vi "SMC_GetError.vi"(8 "error in (no error)":errorcluster) -> (0 "error out":errorcluster, 1 "ErrorText":string, 3 "Answer":string)   [LabVIEW 2015]
uses:
  SMC_SubVIs.llb/SMC_ManagerMode.ctl
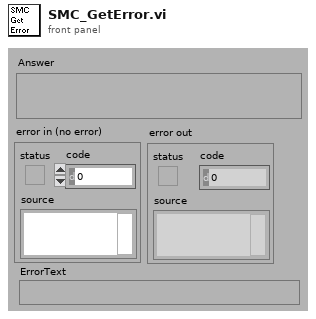
[diagram p1: front panel]
types:
  T1 = typedef "SMC_ManagerMode.ctl" = enum16{"Init", "Get", "SetPosition", "SetStatus", "SetMoving", "SetControllerNr"}
  T2 = typedef "SMC Paras.ctl" = cluster{"VENUS Language":T3, "Number of Axis":u8, "Controller Nr":u8, "Simulation":bool}
  T3 = typedef "VENUSNr.ctl" = enum16{"VENUS 2", "VENUS 1"}
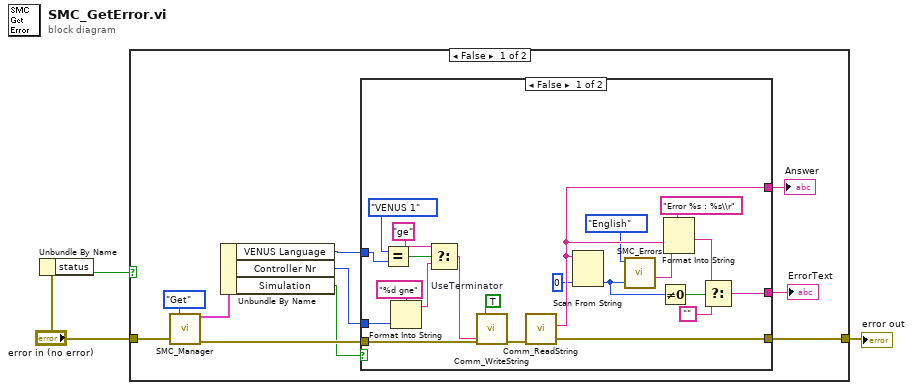
[diagram p0: block diagram]
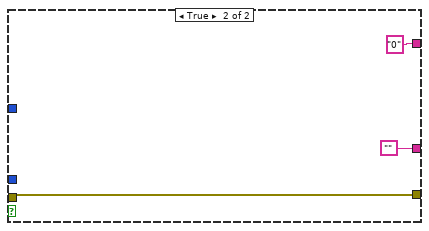
[diagram p2: hidden frame]
diagram:
  n1 = Unbundle By Name("error in (no error)") -> ("status"=w2:bool)
  n2 = case shown="False" w2 {
    tunnel: "error in (no error)" -> [w9 w39]
    tunnel: [w10 w39] -> w1
    frame False {
      n3 = call "SMC_Manager.vi"("Mode"=SMC_ManagerMode."Get", "error in (no error)"=w9) -> ("SMC Parameter Out"=w7:T2, "error out"=w8:errorcluster)  [unwired: 9 in, 3 out]
      n4 = Unbundle By Name(w7) -> ("VENUS Language"=w5:T3, "Controller Nr"=w6:u8, "Simulation"=w4:bool)
      n5 = case shown="False" w4 {
        tunnel: [w35 ""] -> w12
        tunnel: [w34 "0" ("Answer")] -> w11
        tunnel: [w33 w36] -> w10
        tunnel: w8 -> [w32 w36]
        tunnel: w5 -> [w21 _]
        tunnel: w6 -> [w15 _]
        frame False {
          w14 = TRUE  # UseTerminator
          n6 = Equal?(x=enum16{"VENUS 2", "VENUS 1"}."VENUS 1", y=w21) -> (x = y?=w22:bool)
          n7 = Format Into String(format string="%d gne" ("Format String"), w15) -> (resulting string=w16:string)  [unwired: 2 in, 1 out]
          n8 = Select(t="ge" ("string to write"), s=w22, f=w16) -> (s? t:f=w19:string)
          n9 = call "Comm_WriteString.vi"("string to write"=w19, "error in (no error)"=w32, "UseTerminator"=w14) -> ("error out"=w23:errorcluster)  [unwired: 8 in]
          n10 = call "Comm_ReadString.vi"("error in (no error)"=w23) -> ("error out"=w33:errorcluster, "Answer"=w34:string)  [unwired: 9 in]
          n11 = Scan From String(input string=w34, default 1=0) -> (output 1=w25:i32)  [unwired: 3 in, 3 out]
          n12 = call "SMC_Errors.vi"("Error Code"=w25, "Language"=enum16{"Deutsch", "English"}."English") -> ("Answer"=w29:string)  [unwired: 9 in]
          n13 = Not Equal To 0?(x=w25) -> (x != 0?=w26:bool)
          n14 = Format Into String(format string="Error %s : %s\\r", w34, w29) -> (resulting string=w30:string)  [unwired: 2 in, 1 out]
          n15 = Select(t=w30, s=w26, f="") -> (s? t:f=w35:string)
        }
        frame True {
        }
      }
      "Answer" <- w11
      "ErrorText" <- w12
    }
    frame True {
      # "Error, do nothing"
    }
  }
  "error out" <- w1
